vi "Begin.vi"() -> (0 "error out":errorcluster)   [LabVIEW 2013]
doc: "Called before other user functions, this VI is expected to open initial I/O refnums, load in file data, and do all program initialization. Notice that the <B>error out</B> terminal is simply used for data flow. Wiring it to other structures or subVIs ensures that this VI runs first."
uses:
  <vilib>/Rock Robotics/WPI/Camera/WPI_CameraImageSize.ctl
  <vilib>/Rock Robotics/SystemInterfaces/DIO/FPGA_DIOPWMChannel.ctl
  <vilib>/Rock Robotics/WPI/DriverStation/WPI_DriverStationRobotMode2.ctl
  <vilib>/Rock Robotics/WPI/Joystick/WPI_JoystickDeviceEnum.ctl
  <vilib>/Rock Robotics/SystemInterfaces/Typedef/FPGA_TypedefDigitalModule.ctl
  <vilib>/Rock Robotics/SystemInterfaces/DIO/FPGA_DIOChannel.ctl
  <vilib>/Rock Robotics/WPI/Encoder/WPI_EncoderType.ctl
  <vilib>/Rock Robotics/WPI/Camera/WPI_CameraWhite Balance Values.ctl
  <vilib>/Rock Robotics/WPI/Camera/WPI_CameraExposure Values.ctl
  <vilib>/Rock Robotics/WPI/Camera/WPI_CameraFrameRate.ctl
  <vilib>/Rock Robotics/WPI/Solenoid/WPI_SolenoidChannel.ctl
  <vilib>/Rock Robotics/SystemInterfaces/Typedef/FPGA_TypedefSolenoidModule.ctl
  <vilib>/Rock Robotics/SystemInterfaces/Typedef/FPGA_TypedefAnalogModule.ctl
  <vilib>/Rock Robotics/SystemInterfaces/AI/FPGA_AIChannel.ctl
  <vilib>/Rock Robotics/SystemInterfaces/DIO/FPGA_DIORelayChannel.ctl
  <vilib>/Rock Robotics/WPI/RobotDrive/WPI_RobotDriveOpen2MotorWithTalon.vi
  Robot Global Data.vi
  <vilib>/Rock Robotics/WPI/Counter/WPI_CounterDigitalInputToDigitalSource.vi
  <vilib>/Rock Robotics/WPI/Solenoid/WPI_SolenoidOpenDouble.vi
  <vilib>/Rock Robotics/WPI/MotorControl/WPI_MotorControlOpen Talon.vi
  <vilib>/Rock Robotics/WPI/Compressor/WPI_CompressorGetSetRefNum.vi
panel:
  in  "Image Size 2":T1=enum."160x120"
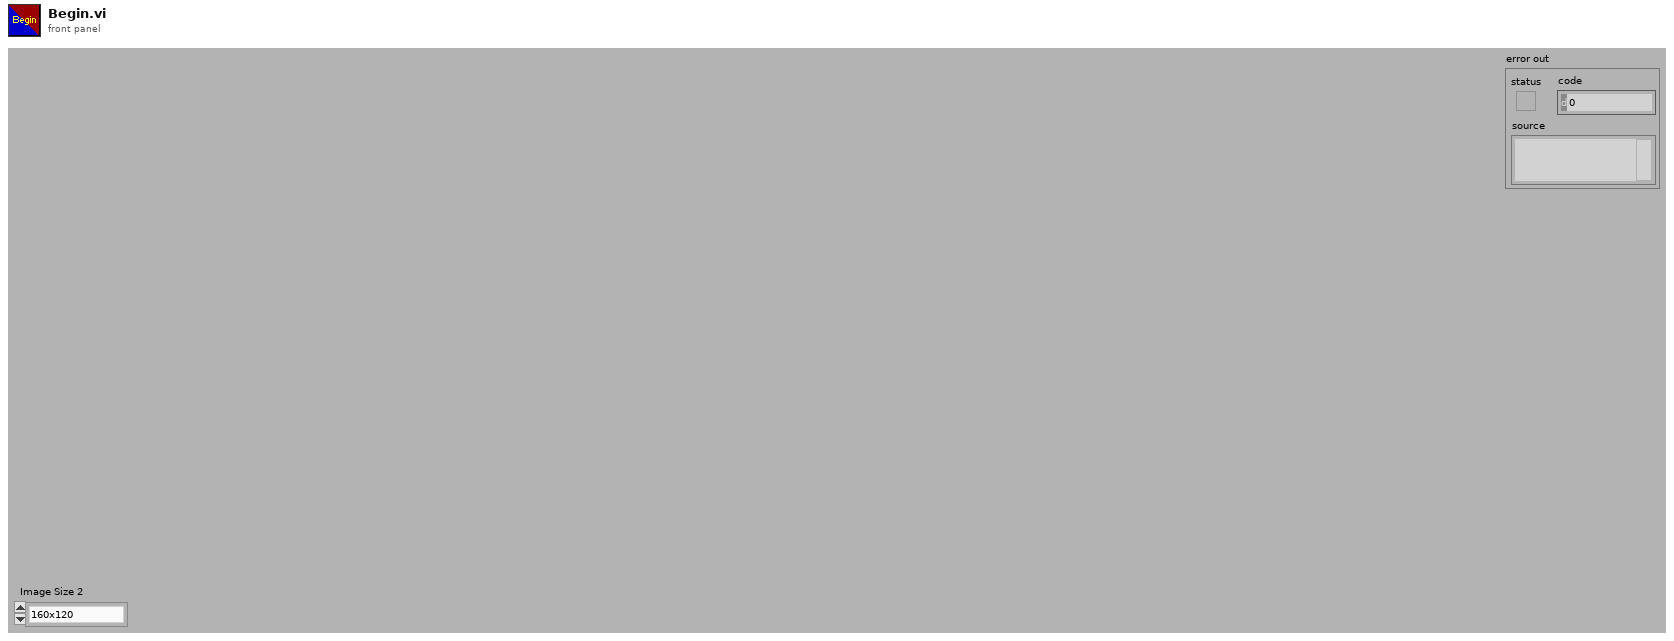
[diagram p1: front panel]
types:
  T1 = typedef "WPI_CameraImageSize.ctl" = enum16{"640x480", "320x240", "160x120"}
  T2 = typedef "FPGA_TypedefDigitalModule.ctl" = enum16{"Digital Module 1", "Digital Module 2"}
  T3 = typedef "FPGA_DIORelayChannel.ctl" = enum8{"Relay 1", "Relay 2", "Relay 3", "Relay 4", "Relay 5", "Relay 6", "Relay 7", "Relay 8", "Invalid"}
  T4 = typedef "FPGA_DIOChannel.ctl" = enum8{"DIO 1", "DIO 2", "DIO 3", "DIO 4", "DIO 5", "DIO 6", "DIO 7", "DIO 8", "DIO 9", "DIO 10", "DIO 11", "DIO 12", "DIO 13", "DIO 14", "Invalid"}
  T5 = typedef "FPGA_DIOPWMChannel.ctl" = enum8{"PWM 1", "PWM 2", "PWM 3", "PWM 4", "PWM 5", "PWM 6", "PWM 7", "PWM 8", "PWM 9", "PWM 10", "Invalid"}
  T6 = typedef "FPGA_AIChannel.ctl" = enum8{"AI 1", "AI 2", "AI 3", "AI 4", "AI 5", "AI 6", "AI 7", "AI 8", "Invalid"}
  T7 = typedef "FPGA_TypedefAnalogModule.ctl" = enum16{"Analog Module 1", "Analog Module 2"}
  T8 = typedef "WPI_SolenoidChannel.ctl" = enum8{"Solenoid 1", "Solenoid 2", "Solenoid 3", "Solenoid 4", "Solenoid 5", "Solenoid 6", "Solenoid 7", "Solenoid 8", "Invalid"}
  T9 = typedef "FPGA_TypedefSolenoidModule.ctl" = enum16{"Solenoid Module 1", "Solenoid Module 2"}
  T10 = typedef "WPI_EncoderType.ctl" = enum16{"1x", "2x", "4x"}
  T11 = typedef "WPI_CameraFrameRate.ctl" = u32
  T12 = typedef "WPI_CameraExposure Values.ctl" = enum16{"Auto", "Flicker-free 50 Hz", "Flicker-free 60 Hz", "Hold current"}
  T13 = typedef "WPI_CameraWhite Balance Values.ctl" = enum16{"Auto", "Fixed indoor", "Fixed outdoor 1", "Fixed outdoor 2", "Fixed fluorescent 1", "Fixed fluorescent 2", "Hold current"}
  T14 = typedef "WPI_JoystickDeviceEnum.ctl" = enum16{"USB 1", "USB 2", "USB 3", "USB 4", "Kinect 1", "Kinect 2"}
  T15 = typedef "WPI_DriverStationRobotMode2.ctl" = enum16{"Autonomous Disabled", "Autonomous Enabled", "Teleop Disabled", "Teleop Enabled", "Timeout", "Finish", "Test Disabled", "Test Enabled"}
  T16 = typedef "WPI_JoystickDevRef.ctl" = cluster{"Device":T14}
  T17 = typedef "WPI_DigitalInputDevRef.ctl" = cluster{"DevStatus":errorcluster, "DIO Channel":T4, "Digital Module":T2}
  T18 = typedef "WPI_SolenoidDevRef.ctl" = cluster{"DevStatus":errorcluster, "Solenoid Module":T9, "Forward Solenoid Channel":T8, "Reverse Solenoid Channel":T8}
  T19 = typedef "WPI_AnalogChannelDevRef.ctl" = cluster{"DevStatus":errorcluster, "Analog Module":T7, "Analog Channel":T6}
  T20 = typedef "FPGA_CounterEncoderSourceConvertionLVSourceType.ctl" = cluster{"DevStatus":errorcluster, "AnalogTriggerMode?":bool, "DigitalMode":cluster{"Digital Module":T2, "DIO Channel":T21}, "AnalogTriggerMode":cluster{"AnalogTriggerIndex":T22, "OutputType":T23}}
  T21 = typedef "FPGA_DIODigitalSourceChannel.ctl" = enum8{"DIO 1", "DIO 2", "DIO 3", "DIO 4", "DIO 5", "DIO 6", "DIO 7", "DIO 8", "DIO 9", "DIO 10", "DIO 11", "DIO 12", "DIO 13", "DIO 14", "Disabled"}
  T22 = typedef "FPGA_AnalogTriggerIndex.ctl" = enum8{"Trig 0", "Trig 1", "Trig 2", "Trig 3", "Trig 4", "Trig 5", "Trig 6", "Trig 7", "Invalid"}
  T23 = typedef "FPGA_AnalogTriggerOutType.ctl" = enum16{"InWindow", "TriggerState", "Rising", "Falling"}
  T24 = typedef "WPI_EncoderDevRef.ctl" = cluster{"DevStatus":errorcluster, "EncoderIndex":T25, "CounterIndex":T26, "DistancePerCount":dbl, "Decoding Type":T10}
  T25 = typedef "FPGA_EncoderIdx.ctl" = enum8{"Enc 0", "Enc 1", "Enc 2", "Enc 3", "Invalid"}
  T26 = typedef "FPGA_CounterCtrSystemIndex.ctl" = enum8{"Ctr 0", "Ctr 1", "Ctr 2", "Ctr 3", "Ctr 4", "Ctr 5", "Ctr 6", "Ctr 7", "Invalid"}
  T27 = typedef "WPI_CompressorDevRef.ctl" = cluster{"DevStatus":errorcluster, "DigitalInputDevRef":T17, "RelayDevRef":T28}
  T28 = typedef "WPI_RelayDevRef.ctl" = cluster{"DevStatus":errorcluster, "Relay Channel":T3, "Digital Module":T2, "Relay Direction":T29}
  T29 = typedef "WPI_RelayDirection.ctl" = enum16{"Both directions", "Forward only", "Reverse only"}
  T30 = typedef "WPI_RobotDriveDevRef.ctl" = cluster{"DevStatus":errorcluster, "Motors[]":T31[], "Square Inputs":bool, "Max Output":dbl, "Isochronous":bool}
  T31 = typedef "WPI_MotorControlDeviceRef.ctl" = cluster{"DeviceStatus":errorcluster, "Type":enum16{"PWM", "CAN"}, "PWM":cluster{"Digital Module":T2, "PWM Channel":T5, "DeadBand":T32}, "CAN":cluster{"Device Number":u8, "Control Mode":T33, "Semaphore":T34, "Max Vout":dbl}, "Invert":bool, "TransformRef":T35, "InvTransformRef":T35}
  T32 = typedef "WPI_PWMDeadband.ctl" = cluster{"Name":string, "maxPositivePwm":i32, "minPositivePwm":i32, "centerPwm":i32, "maxNegativePwm":i32, "minNegativePwm":i32, "angularRange":u16}
  T33 = typedef "WPI_CANJaguar_ControlMode.ctl" = enum8{"Percent VBus", "Current", "Speed", "Position", "Voltage"}
  T34 = typedef "Semaphore RefNum" = refnum<k1>
  T35 = typedef "WPI_PWMTransform_ConPane.ctl" = refnum<vi>
  T36 = typedef "WPI_CameraDevRef.ctl" = cluster{"Camera Address":string, "CameraStatus":errorcluster, "Acquire Image Notifier":refnum<notifier>}
  T37 = typedef "WPI_ServoDeviceRef.ctl" = cluster{"DeviceStatus":errorcluster, "Digital Module":T2, "PWM Channel":T5, "DeadBand":T32}
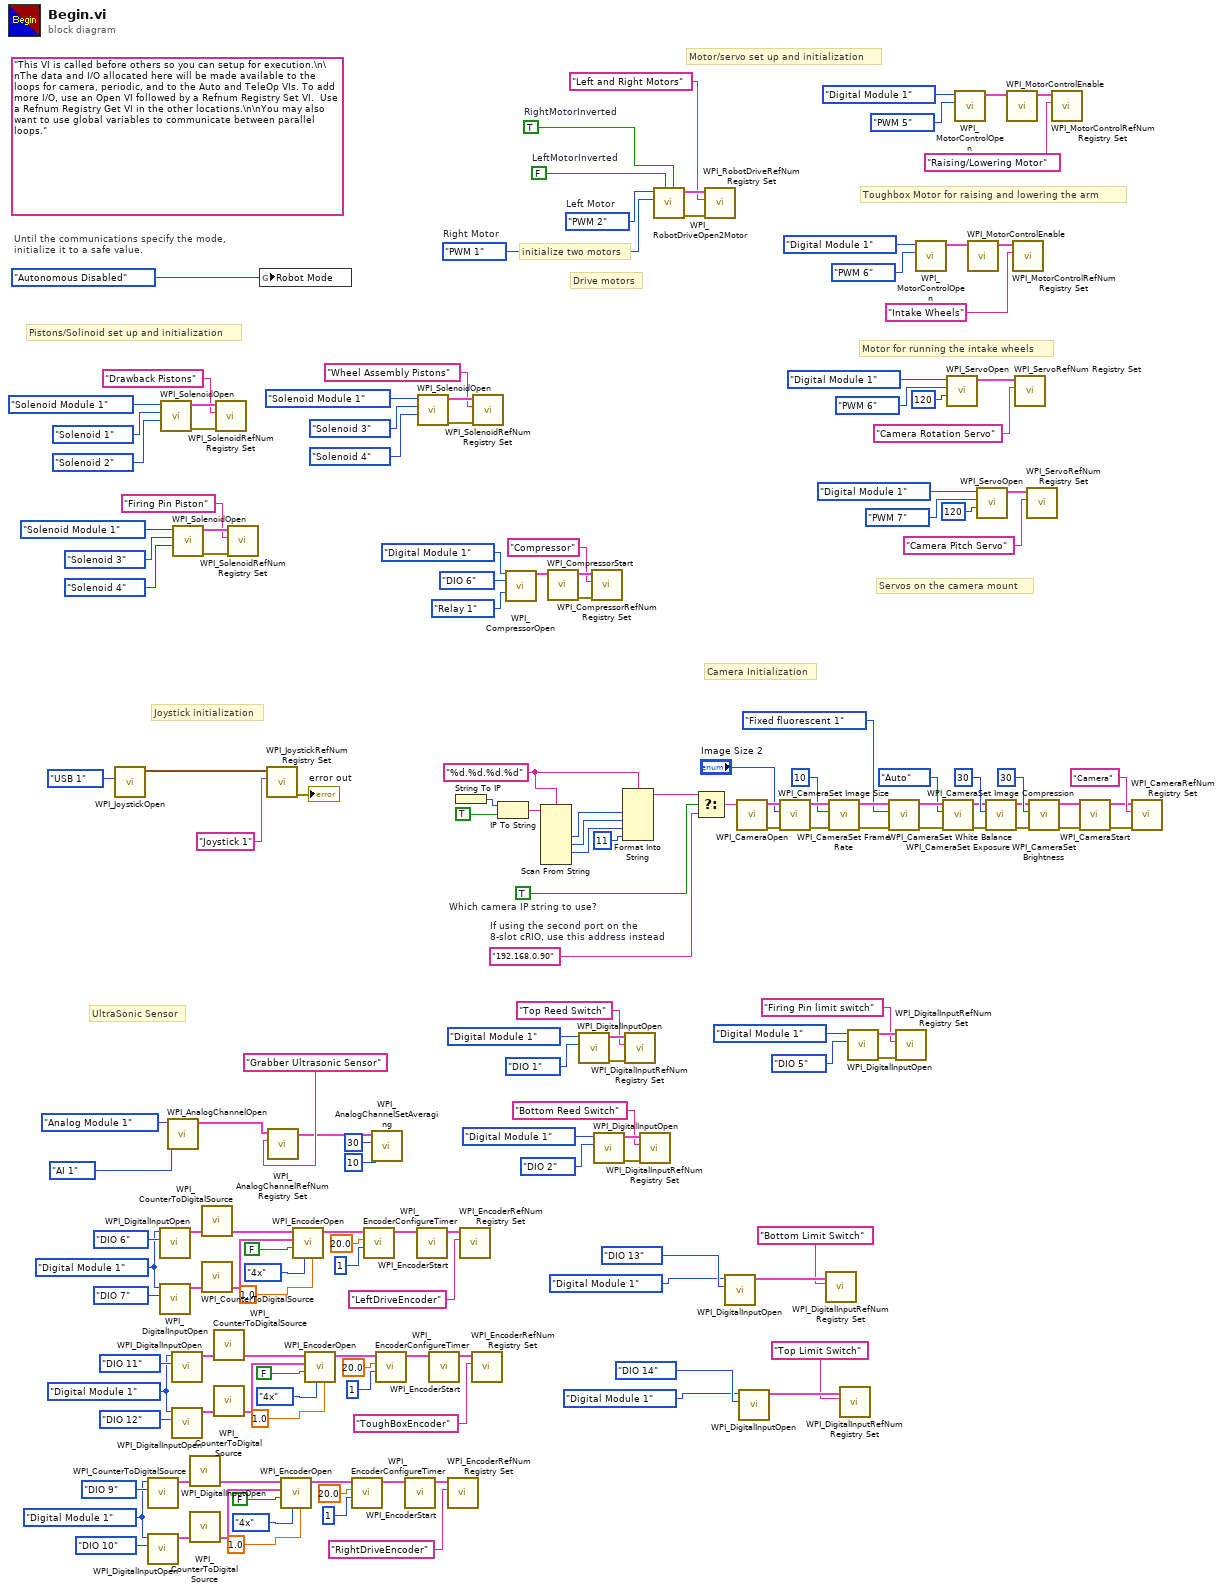
[diagram p0: block diagram]
diagram:
  w51 = FPGA_TypedefDigitalModule."Digital Module 1" ("DIO Module")
  w96 = TRUE  # Which camera IP string to use?
  w100 = "%d.%d.%d.%d" ("format string")
  w97 = "192.168.0.90"  # If using the second port on the 8-slot cRIO, use this address instead
  w129 = FPGA_TypedefDigitalModule."Digital Module 1" ("DIO Module")
  w145 = FPGA_TypedefDigitalModule."Digital Module 1" ("DIO Module")
  (unwired) "This VI is called before others so you can setup for execution.\n\nThe data and I/O allocated here will be made available to the loops for camera, periodic, and to the Auto and TeleOp VIs. To add more I/O, use an Open VI followed by a Refnum Registry Set VI.  Use a Refnum Registry Get VI in the other locations.\n\nYou may also want to use global variables to communicate between parallel loops."
  w164 = FPGA_DIOPWMChannel."PWM 1"  # Right Motor
  w165 = FPGA_DIOPWMChannel."PWM 2"  # Left Motor
  w169 = FALSE  # LeftMotorInverted
  w170 = TRUE  # RightMotorInverted
  # "UltraSonic Sensor"
  # "Servos on the camera mount"
  # "Motor for running the intake wheels"
  # "Pistons/Solinoid set up and initialization"
  # "Toughbox Motor for raising and lowering the arm"
  # "Drive motors"
  # "Motor/servo set up and initialization"
  # "Camera Initialization"
  # "Joystick initialization"
  # "Until the communications specify the mode,\ninitialize it to a safe value."
  # "initialize two motors"
  n1 = call <vilib>:"WPI_JoystickOpen.vi"("JoystickDevice"=WPI_JoystickDeviceEnum."USB 1") -> ("JoystickDevRef"=w161:T16)  [unwired: 10 in]
  n2 = call <vilib>:"WPI_DigitalInputOpen.vi"("DIO Channel"=FPGA_DIOChannel."DIO 9" ("A Channel"), "Digital Module (Module 1)"=w129) -> ("DigitalInputDevRef"=w140:T17)  [unwired: 1 in, 8 out]
  n3 = call <vilib>:"WPI_DigitalInputOpen.vi"("DIO Channel"=FPGA_DIOChannel."DIO 10" ("B Channel"), "Digital Module (Module 1)"=w129) -> ("DigitalInputDevRef"=w141:T17)  [unwired: 1 in, 8 out]
  n4 = call <vilib>:"WPI_DigitalInputOpen.vi"("DIO Channel"=FPGA_DIOChannel."DIO 6" ("A Channel"), "Digital Module (Module 1)"=w145) -> ("DigitalInputDevRef"=w156:T17)  [unwired: 1 in, 8 out]
  n5 = call <vilib>:"WPI_DigitalInputOpen.vi"("DIO Channel"=FPGA_DIOChannel."DIO 7" ("B Channel"), "Digital Module (Module 1)"=w145) -> ("DigitalInputDevRef"=w157:T17)  [unwired: 1 in, 8 out]
  n6 = call-poly <vilib>:"WPI_SolenoidOpen.vi"("Reverse Solenoid Channel"=WPI_SolenoidChannel."Solenoid 2" ("Extend Solenoid Channel"), "Forward Solenoid Channel"=WPI_SolenoidChannel."Solenoid 1" ("Retract Solenoid Channel"), "Solenoid Module (Module 1)"=FPGA_TypedefSolenoidModule."Solenoid Module 1" ("Solenoid Module")) -> ("error out"=w83:errorcluster, "SolenoidDevRef"=w82:T18)  [unwired: 1 in, 6 out]
  n7 = call <vilib>:"WPI_AnalogChannelOpen.vi"("Analog Channel"=FPGA_AIChannel."AI 1", "Analog Module (Module 1)"=FPGA_TypedefAnalogModule."Analog Module 1") -> ("AIDeviceRef"=w36:T19)  [unwired: 8 in, 1 out]
  n8 = call <vilib>:"WPI_DigitalInputOpen.vi"("DIO Channel"=FPGA_DIOChannel."DIO 11" ("A Channel"), "Digital Module (Module 1)"=w51) -> ("DigitalInputDevRef"=w62:T17)  [unwired: 1 in, 8 out]
  n9 = call <vilib>:"WPI_DigitalInputOpen.vi"("DIO Channel"=FPGA_DIOChannel."DIO 12" ("B Channel"), "Digital Module (Module 1)"=w51) -> ("DigitalInputDevRef"=w63:T17)  [unwired: 1 in, 8 out]
  n10 = call-poly <vilib>:"WPI_SolenoidOpen.vi"("Reverse Solenoid Channel"=WPI_SolenoidChannel."Solenoid 4" ("Extend Solenoid Channel"), "Forward Solenoid Channel"=WPI_SolenoidChannel."Solenoid 3" ("Retract Solenoid Channel"), "Solenoid Module (Module 1)"=FPGA_TypedefSolenoidModule."Solenoid Module 1" ("Solenoid Module")) -> ("error out"=w77:errorcluster, "SolenoidDevRef"=w76:T18)  [unwired: 1 in, 6 out]
  n11 = call-poly <vilib>:"WPI_CounterToDigitalSource.vi"("DigitalInputDevRef"=w140) -> ("Digital Source"=w139:T20)  [unwired: 6 out]
  n12 = call-poly <vilib>:"WPI_CounterToDigitalSource.vi"("DigitalInputDevRef"=w141) -> ("Digital Source"=w142:T20)  [unwired: 6 out]
  n13 = call-poly <vilib>:"WPI_CounterToDigitalSource.vi"("DigitalInputDevRef"=w156) -> ("Digital Source"=w155:T20)  [unwired: 6 out]
  n14 = call-poly <vilib>:"WPI_CounterToDigitalSource.vi"("DigitalInputDevRef"=w157) -> ("Digital Source"=w158:T20)  [unwired: 6 out]
  n15 = call-poly <vilib>:"WPI_CounterToDigitalSource.vi"("DigitalInputDevRef"=w62) -> ("Digital Source"=w61:T20)  [unwired: 6 out]
  n16 = call-poly <vilib>:"WPI_CounterToDigitalSource.vi"("DigitalInputDevRef"=w63) -> ("Digital Source"=w64:T20)  [unwired: 6 out]
  n17 = call <vilib>:"WPI_SolenoidRefNum Registry Set.vi"("error in (no error)"=w83, "refnum name"="Drawback Pistons", "SolenoidDevRef"=w82) -> ()  [unwired: 7 in, 2 out]
  n18 = call <vilib>:"WPI_SolenoidRefNum Registry Set.vi"("error in (no error)"=w77, "refnum name"="Firing Pin Piston", "SolenoidDevRef"=w76) -> ()  [unwired: 7 in, 2 out]
  n19 = global write "Robot Global Data.vi" "Robot Mode"(WPI_DriverStationRobotMode2."Autonomous Disabled" ("Robot Mode")) -> ()
  n20 = call <vilib>:"WPI_JoystickRefNum Registry Set.vi"("refnum name"="Joystick 1", "JoystickDevRef"=w161) -> ("error out"=→"error out":errorcluster)  [unwired: 8 in, 1 out]
  n21 = call <vilib>:"WPI_AnalogChannelRefNum Registry Set.vi"("refnum name"="Grabber Ultrasonic Sensor", "AIDeviceRef"=w36) -> ("AIDeviceRef"=w34:T19)  [unwired: 8 in, 1 out]
  n22 = call <vilib>:"WPI_EncoderOpen.vi"("DistancePerCount"=1.0, "Decoding Type"=WPI_EncoderType."4x", "Invert Direction (False)"=FALSE ("Invert Direction"), "BSource"=w142, "ASource"=w139) -> ("EncoderDevRef"=w132:T24)  [unwired: 3 in, 3 out]
  n23 = call <vilib>:"WPI_EncoderOpen.vi"("DistancePerCount"=1.0, "Decoding Type"=WPI_EncoderType."4x", "Invert Direction (False)"=FALSE ("Invert Direction"), "BSource"=w158, "ASource"=w155) -> ("EncoderDevRef"=w148:T24)  [unwired: 3 in, 3 out]
  n24 = call <vilib>:"WPI_EncoderOpen.vi"("DistancePerCount"=1.0, "Decoding Type"=WPI_EncoderType."4x", "Invert Direction (False)"=FALSE ("Invert Direction"), "BSource"=w64, "ASource"=w61) -> ("EncoderDevRef"=w54:T24)  [unwired: 3 in, 3 out]
  n25 = call <vilib>:"WPI_EncoderConfigureTimer.vi"("Number Samples to Average"=u8 1, "Minimum Rate"=20.0, "EncoderDevRef"=w132) -> ("EncoderDevRef"=w133:T24)  [unwired: 1 in, 7 out]
  n26 = call <vilib>:"WPI_EncoderConfigureTimer.vi"("Number Samples to Average"=u8 1, "Minimum Rate"=20.0, "EncoderDevRef"=w148) -> ("EncoderDevRef"=w149:T24)  [unwired: 1 in, 7 out]
  n27 = call <vilib>:"WPI_AnalogChannelSetAveraging.vi"("OversampleBits"=u8 10, "AverageBits"=u8 30, "AIDeviceRef"=w34) -> ()  [unwired: 7 in, 2 out]
  n28 = call <vilib>:"WPI_EncoderConfigureTimer.vi"("Number Samples to Average"=u8 1, "Minimum Rate"=20.0, "EncoderDevRef"=w54) -> ("EncoderDevRef"=w55:T24)  [unwired: 1 in, 7 out]
  n29 = call <vilib>:"WPI_EncoderStart.vi"("EncoderDevRef"=w133) -> ("EncoderDevRef"=w128:T24)  [unwired: 1 in, 9 out]
  n30 = call <vilib>:"WPI_EncoderStart.vi"("EncoderDevRef"=w149) -> ("EncoderDevRef"=w144:T24)  [unwired: 1 in, 9 out]
  n31 = call-poly <vilib>:"WPI_SolenoidOpen.vi"("Reverse Solenoid Channel"=WPI_SolenoidChannel."Solenoid 4" ("Extend Solenoid Channel"), "Forward Solenoid Channel"=WPI_SolenoidChannel."Solenoid 3" ("Retract Solenoid Channel"), "Solenoid Module (Module 1)"=FPGA_TypedefSolenoidModule."Solenoid Module 1" ("Solenoid Module")) -> ("error out"=w41:errorcluster, "SolenoidDevRef"=w40:T18)  [unwired: 1 in, 6 out]
  n32 = call <vilib>:"WPI_EncoderStart.vi"("EncoderDevRef"=w55) -> ("EncoderDevRef"=w50:T24)  [unwired: 1 in, 9 out]
  n33 = call <vilib>:"WPI_EncoderRefNum Registry Set.vi"("refnum name"="RightDriveEncoder", "EncoderDevRef"=w128) -> ()  [unwired: 8 in, 2 out]
  n34 = String To IP() -> (0:w107:u32)  [unwired: 1 in]
  n35 = call <vilib>:"WPI_EncoderRefNum Registry Set.vi"("refnum name"="LeftDriveEncoder", "EncoderDevRef"=w144) -> ()  [unwired: 8 in, 2 out]
  n36 = call <vilib>:"WPI_EncoderRefNum Registry Set.vi"("refnum name"="ToughBoxEncoder", "EncoderDevRef"=w50) -> ()  [unwired: 8 in, 2 out]
  n37 = call <vilib>:"WPI_SolenoidRefNum Registry Set.vi"("error in (no error)"=w41, "refnum name"="Wheel Assembly Pistons", "SolenoidDevRef"=w40) -> ()  [unwired: 7 in, 2 out]
  n38 = IP To String(1:TRUE ("dot notation? (F)"), 2:w107) -> (0:w105:string)
  n39 = call <vilib>:"WPI_CompressorOpen.vi"("Pressure Switch Digital Module (Module 1)"=FPGA_TypedefDigitalModule."Digital Module 1" ("Switch and Relay Module"), "Pressure Switch DIO Channel"=FPGA_DIOChannel."DIO 6" ("Pressure Switch Channel"), "Relay Channel"=FPGA_DIORelayChannel."Relay 1" ("RelayChannel")) -> ("CompressorDevRef"=w5:T27)  [unwired: 2 in, 10 out]
  n40 = Scan From String(format string=w100, input string=w105) -> (output 1=w104:i32, output 2=w103:i32, output 3=w102:i32)  [unwired: 7 in, 3 out]
  n41 = call <vilib>:"WPI_CompressorStart.vi"("CompressorDevRef"=w5) -> ("error out"=w4:errorcluster, "CompressorDevRef"=w3:T27)  [unwired: 1 in, 8 out]
  n42 = call <vilib>:"WPI_DigitalInputOpen.vi"("DIO Channel"=FPGA_DIOChannel."DIO 1" ("Limit Switch Channel"), "Digital Module (Module 1)"=FPGA_TypedefDigitalModule."Digital Module 1" ("Switch and Relay Module")) -> ("error out"=w86:errorcluster, "DigitalInputDevRef"=w85:T17)  [unwired: 1 in, 7 out]
  n43 = call <vilib>:"WPI_CompressorRefNum Registry Set.vi"("error in (no error)"=w4, "refnum name"="Compressor", "CompressorDevRef"=w3) -> ()  [unwired: 7 in, 2 out]
  n44 = call <vilib>:"WPI_DigitalInputOpen.vi"("DIO Channel"=FPGA_DIOChannel."DIO 2" ("Limit Switch Channel"), "Digital Module (Module 1)"=FPGA_TypedefDigitalModule."Digital Module 1" ("Switch and Relay Module")) -> ("error out"=w72:errorcluster, "DigitalInputDevRef"=w71:T17)  [unwired: 1 in, 7 out]
  n45 = Format Into String(format string=w100, w104, w103, w102, 11 ("Compression")) -> (resulting string=w98:string)  [unwired: 2 in, 1 out]
  n46 = call <vilib>:"WPI_DigitalInputRefNum Registry Set.vi"("error in (no error)"=w86, "refnum name"="Top Reed Switch", "DigitalInputDevRef"=w85) -> ()  [unwired: 7 in, 2 out]
  n47 = call <vilib>:"WPI_DigitalInputRefNum Registry Set.vi"("error in (no error)"=w72, "refnum name"="Bottom Reed Switch", "DigitalInputDevRef"=w71) -> ()  [unwired: 7 in, 2 out]
  n48 = call-poly <vilib>:"WPI_RobotDriveOpen2Motor.vi"("Right Motor Inverted"=w170, "Left Motor Inverted"=w169, "Right Motor"=w164, "Left Motor"=w165) -> ("error out"=w166:errorcluster, "RobotDriveDevRef"=w168:T30)  [unwired: 1 in, 5 out]
  n49 = Select(t=w98, s=w96, f=w97) -> (s? t:f=w99:string)
  n50 = call <vilib>:"WPI_RobotDriveRefNum Registry Set.vi"("error in (no error)"=w166, "refnum name"="Left and Right Motors", "RobotDriveDevRef"=w168) -> ()  [unwired: 9 out]
  n51 = call <vilib>:"WPI_DigitalInputOpen.vi"("DIO Channel"=FPGA_DIOChannel."DIO 13" ("A Channel"), "Digital Module (Module 1)"=FPGA_TypedefDigitalModule."Digital Module 1" ("DIO Module")) -> ("DigitalInputDevRef"=w46:T17)  [unwired: 8 in, 1 out]
  n52 = call <vilib>:"WPI_CameraOpen.vi"("Camera Address"=w99) -> ("error out"=w117:errorcluster, "CameraDevRef"=w118:T36)  [unwired: 1 in, 8 out]
  n53 = call <vilib>:"WPI_DigitalInputOpen.vi"("DIO Channel"=FPGA_DIOChannel."DIO 14" ("A Channel"), "Digital Module (Module 1)"=FPGA_TypedefDigitalModule."Digital Module 1" ("DIO Module")) -> ("DigitalInputDevRef"=w29:T17)  [unwired: 8 in, 1 out]
  n54 = call <vilib>:"WPI_CameraSet Image Size.vi"("error in (no error)"=w117, "Image Size"="Image Size 2", "CameraDevRef"=w118) -> ("error out"=w116:errorcluster, "CameraDevRef Out"=w119:T36)  [unwired: 7 out]
  n55 = call <vilib>:"WPI_DigitalInputRefNum Registry Set.vi"("refnum name"="Bottom Limit Switch", "DigitalInputDevRef"=w46) -> ()  [unwired: 8 in, 2 out]
  n56 = call <vilib>:"WPI_CameraSet Frame Rate.vi"("error in (no error)"=w116, "Frame Rate (fps)"=T11 10, "CameraDevRef"=w119) -> ("error out"=w115:errorcluster, "CameraDevRef Out"=w121:T36)  [unwired: 7 out]
  n57 = call <vilib>:"WPI_DigitalInputRefNum Registry Set.vi"("refnum name"="Top Limit Switch", "DigitalInputDevRef"=w29) -> ()  [unwired: 8 in, 2 out]
  n58 = call <vilib>:"WPI_DigitalInputOpen.vi"("DIO Channel"=FPGA_DIOChannel."DIO 5", "Digital Module (Module 1)"=FPGA_TypedefDigitalModule."Digital Module 1") -> ("error out"=w66:errorcluster, "DigitalInputDevRef"=w67:T17)  [unwired: 1 in, 7 out]
  n59 = call <vilib>:"WPI_CameraSet White Balance.vi"("error in (no error)"=w115, "White Balance"=WPI_CameraWhite_Balance_Values."Fixed fluorescent 1", "CameraDevRef"=w121) -> ("error out"=w114:errorcluster, "CameraDevRef Out"=w120:T36)  [unwired: 7 out]
  n60 = call <vilib>:"WPI_DigitalInputRefNum Registry Set.vi"("error in (no error)"=w66, "refnum name"="Firing Pin limit switch", "DigitalInputDevRef"=w67) -> ()  [unwired: 7 in, 2 out]
  n61 = call-poly <vilib>:"WPI_MotorControlOpen.vi"("PWM Channel"=FPGA_DIOPWMChannel."PWM 6" ("Left Motor"), "Digital Module (Module 1)"=enum16{"Digital Module 1"}."Digital Module 1") -> ("MotorControlDeviceRef"=w19:T31)  [unwired: 8 in, 1 out]
  n62 = call <vilib>:"WPI_CameraSet Exposure.vi"("error in (no error)"=w114, "Exposure"=WPI_CameraExposure_Values."Auto", "CameraDevRef"=w120) -> ("error out"=w113:errorcluster, "CameraDevRef Out"=w123:T36)  [unwired: 7 out]
  n63 = call <vilib>:"WPI_ServoOpen.vi"("Angular Range"=u16 120, "PWM Channel"=FPGA_DIOPWMChannel."PWM 6", "Digital Module (Module 1)"=FPGA_TypedefDigitalModule."Digital Module 1") -> ("ServoDeviceRef"=w10:T37)  [unwired: 7 in, 1 out]
  n64 = call-poly <vilib>:"WPI_MotorControlOpen.vi"("PWM Channel"=FPGA_DIOPWMChannel."PWM 5" ("Left Motor"), "Digital Module (Module 1)"=enum16{"Digital Module 1"}."Digital Module 1") -> ("MotorControlDeviceRef"=w25:T31)  [unwired: 8 in, 1 out]
  n65 = call <vilib>:"WPI_MotorControlEnable.vi"("CAN Jaguar Ref"=w19) -> ("CAN Jaguar Ref Out"=w18:T31)  [unwired: 9 in, 1 out]
  n66 = call <vilib>:"WPI_ServoOpen.vi"("Angular Range"=u16 120, "PWM Channel"=FPGA_DIOPWMChannel."PWM 7", "Digital Module (Module 1)"=FPGA_TypedefDigitalModule."Digital Module 1") -> ("ServoDeviceRef"=w11:T37)  [unwired: 7 in, 1 out]
  n67 = call <vilib>:"WPI_CameraSet Image Compression.vi"("error in (no error)"=w113, "Compression"=30, "CameraDevRef"=w123) -> ("error out"=w112:errorcluster, "CameraDevRef Out"=w122:T36)  [unwired: 7 out]
  n68 = call <vilib>:"WPI_MotorControlEnable.vi"("CAN Jaguar Ref"=w25) -> ("CAN Jaguar Ref Out"=w24:T31)  [unwired: 9 in, 1 out]
  n69 = call <vilib>:"WPI_MotorControlRefNum Registry Set.vi"("refnum name"="Intake Wheels", "MotorControlDevRef"=w18) -> ()  [unwired: 8 in, 2 out]
  n70 = call <vilib>:"WPI_ServoRefNum Registry Set.vi"("refnum name"="Camera Rotation Servo", "ServoDeviceRef"=w10) -> ()  [unwired: 8 in, 2 out]
  n71 = call <vilib>:"WPI_ServoRefNum Registry Set.vi"("refnum name"="Camera Pitch Servo", "ServoDeviceRef"=w11) -> ()  [unwired: 8 in, 2 out]
  n72 = call <vilib>:"WPI_CameraSet Brightness.vi"("error in (no error)"=w112, "Brightness"=30, "CameraDevRef"=w122) -> ("error out"=w95:errorcluster, "CameraDevRef Out"=w94:T36)  [unwired: 7 out]
  n73 = call <vilib>:"WPI_MotorControlRefNum Registry Set.vi"("refnum name"="Raising/Lowering Motor", "MotorControlDevRef"=w24) -> ()  [unwired: 8 in, 2 out]
  n74 = call <vilib>:"WPI_CameraStart.vi"("error in (no error)"=w95, "CameraDevRef"=w94) -> ("error out"=w93:errorcluster, "CameraDevRef Out"=w92:T36)  [unwired: 8 in]
  n75 = call <vilib>:"WPI_CameraRefNum Registry Set.vi"("error in (no error)"=w93, "refnum name"="Camera", "CameraDevRef"=w92) -> ()  [unwired: 9 out]
